vi "SGUI Set Multiple Values and Uncertainties to Strings by Label.vi"(0 "labels (empty)":string, 1 "values (empty)":dbl[](array[numeric]), 2 "uncertainties (empty)":dbl[](array[numeric]), 3 "unit (empty)":string, 5 "Add SI prefix (true)":bool=TRUE, 7 "error in":errorcluster) -> (4 "assigned control refs":refnum<vi>[](array[refnum]), 8 "error out":errorcluster)   [LabVIEW 2013, in "varilib.lvlib"]
doc: "This VI sets '(value ± uncerainty) unit' into multiple string controls defined by control labels (must be registered first by calling 'SGUI Register Controls'). The formatter also does SI prefix scaling which can be optionally disabled (mostly for unitless quantities). It automatically formats the value and uncertainty to two significant digits of uncertainty. If unit is assigned it will append it after the value and uncertainty. If multiple string control labels are assigned and just one number it will assign the number to all of them. If no value is assigned it will assign empty strings. It will generate error if control not found or has ivalid type but it ignores input errors (executes anyway)."
uses:
  varilib.lvlib
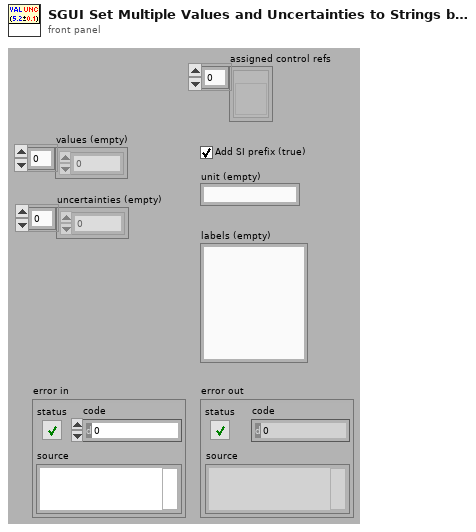
[diagram p1: front panel]
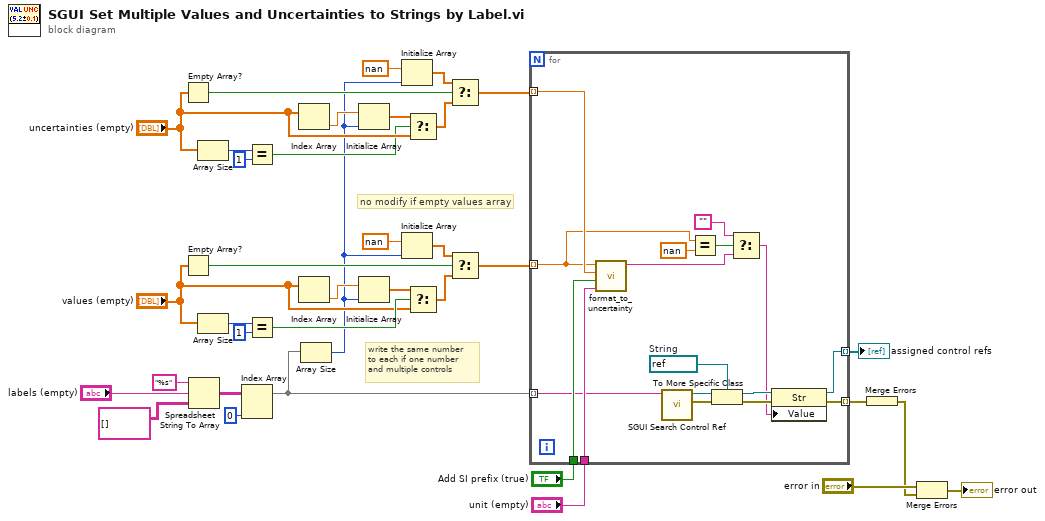
[diagram p0: block diagram]
diagram:
  # "write the same number\nto each if one number\nand multiple controls"
  # "no modify if empty values array"
  n1 = Empty Array?(array="uncertainties (empty)") -> (empty?=w13:bool)
  n2 = Empty Array?(array="values (empty)") -> (empty?=w32:bool)
  n3 = Spreadsheet String To Array(format string="%s", spreadsheet string="labels (empty)", array type (2D Dbl)=string[][] []) -> (array=w33:string[][])  [unwired: 1 in]
  n4 = Array Size(array="uncertainties (empty)") -> (size(s)=w16:i32)
  n5 = Array Size(array="values (empty)") -> (size(s)=w29:i32)
  n6 = Index Array(array=w33, index (col)=0 ("disabled index (col)")) -> (element=w9:string[])  [unwired: 1 in]
  n7 = Equal?(x=w16, y=1) -> (x = y?=w19:bool)
  n8 = Equal?(x=w29, y=1) -> (x = y?=w26:bool)
  n9 = Index Array(array="uncertainties (empty)") -> (element=w21:dbl)  [unwired: 1 in]
  n10 = Index Array(array="values (empty)") -> (element=w24:dbl)  [unwired: 1 in]
  n11 = Array Size(array=w9) -> (size(s)=w12:i32)
  n12 = Initialize Array(w21, w12) -> (w20:dbl[])
  n13 = Initialize Array(w24, w12) -> (w25:dbl[])
  n14 = Initialize Array(nan, w12) -> (w14:dbl[])
  n15 = Initialize Array(nan, w12) -> (w31:dbl[])
  n16 = Select(t=w20, s=w19, f="uncertainties (empty)") -> (s? t:f=w18:dbl[])
  n17 = Select(t=w25, s=w26, f="values (empty)") -> (s? t:f=w27:dbl[])
  n18 = Select(t=w14, s=w13, f=w18) -> (s? t:f=w10:dbl[])
  n19 = Select(t=w31, s=w32, f=w27) -> (s? t:f=w11:dbl[])
  n20 = for {
    tunnel: w11 -> [w43] mode=indexing
    tunnel: w10 -> [w53] mode=indexing
    tunnel: w9 -> [w50] mode=indexing
    tunnel: "Add SI prefix (true)" -> [w52]
    tunnel: "unit (empty)" -> [w51]
    tunnel: [w38] -> w6 mode=indexing
    tunnel: [w37] -> w2 mode=indexing
    w47 = refnum<vi> refnum  # String
    n21 = call "format_to_uncertainty.vi"("unit"=w51, "Add SI prefix (true)"=w52, "uncertainty"=w53, "value"=w43) -> ("string out"=w41:string)  [unwired: 4 in, 3 out]
    n22 = call "SGUI Search Control Ref.vi"("control label (empty)"=w50) -> ("error out"=w49:errorcluster, "control ref out"=w48:refnum<vi>)  [unwired: 8 in, 1 out]
    n23 = Equal?(x=w43, y=nan) -> (x = y?=w44:bool)
    n24 = To More Specific Class(target class=w47, reference=w48, error in=w49) -> (specific class reference=w46:refnum<vi>, error out=w45:errorcluster)
    n25 = Select(t="", s=w44, f=w41) -> (s? t:f=w39:string)
    n26 = property class="Str"(reference=w46, error in=w45, "Value"=w39) -> (reference out=w37:refnum<vi>, error out=w38:errorcluster)
  }
  "assigned control refs" <- w2
  n27 = Merge Errors(w6) -> (w4:errorcluster)
  n28 = Merge Errors("error in", w4) -> (→"error out":errorcluster)
